vi "Measurement Logic.vi"() -> ()   [LabVIEW 2021, in "Efficiency_Channel Ganging.lvlib"]
uses:
  Efficiency_Channel Ganging.lvlib
  Measurement Configuration.ctl
  Measurement Results.ctl
  <vilib>/MeasurementLink/MeasurementLink Measurement Server/Measure Call Context/Measure Call Context.lvclass
  <instrlib>/niDCPower/nidcpower.llb/niDCPower Source Mode.ctl
  <instrlib>/niDCPower/nidcpower.llb/niDCPower Wait For Event - Event.ctl
  <instrlib>/niDCPower/nidcpower.llb/niDCPower Output Function.ctl
  shared subVIs/Triggers and Events/NIDCPower_channel_ganging - Configure Digital Edge Source Trigger.vi
  shared subVIs/Triggers and Events/NIDCPower_channel_ganging - Configure Digital Edge Measure Trigger.vi
  <vilib>/MeasurementLink/MeasurementLink Measurement Server/Measure Call Context/Accessor/Is Canceled.vi
panel:
  out "measure call context out":refnum<class "Measure Call Context.lvclass">
  in  "measure call context in":refnum<class "Measure Call Context.lvclass">
  out "measurement results":T1
  in  "measurement configuration":T2={"Source master resource name"="", "Source slave resource names"=[], "Load master resource name"="", "Load slave resource names"=[], "Source system configuration"=enum."Parallel", "Source start voltage"=6.0, "Source stop voltage"=14.0, "Source voltage sweep points"=4, "Source voltage level range"=20.0, "Source sense"=1009, "Source limit symmetry"=enum."Asymmetric", "Source current limit range"=25.0, "Source current limit low"=-0.6, "Source current limit high"=25.0, "Source transient response"=1038, "Load system configuration"=enum."Parallel", "Load start current"=1.0, "Load stop current"=50.0, "Load current sweep points/points per decade"=10, "Load sweep type"="Logarithmic", "Load current level range"=80.0, "Load sense"=1009, "Load limit symmetry"=enum."Symmetric", "Load voltage limit range"=6.0, "Load voltage limit low"=0.0, "Load voltage limit high"=inf, "Load transient response"=1038, "DUT setup time"=1.0, "Source delay"=0.005, "Aperture time"=0.005} {"Source delay" format="%#_6p"; "DUT setup time" format="%#_6p"; "Load start current" format="%#_6p"; "Source start voltage" format="%#_6p"; "Load sense" items=["Local"=1008, "Remote"=1009]; "Load transient response" items=["Slow"=1041, "Normal"=1038, "Fast"=1039, "Custom"=1042]; "Source sense" items=["Local"=1008, "Remote"=1009]; "Source transient response" items=["Slow"=1041, "Normal"=1038, "Fast"=1039, "Custom"=1042]; "Load voltage limit high" format="%#_6p"; "Load voltage limit low" format="%#_6p"; "Source current limit high" format="%#_6p"; "Source current limit low" format="%#_6p"; "Source current limit range" format="%#_6p"}
  out "error out":errorcluster
  in  "error in":errorcluster
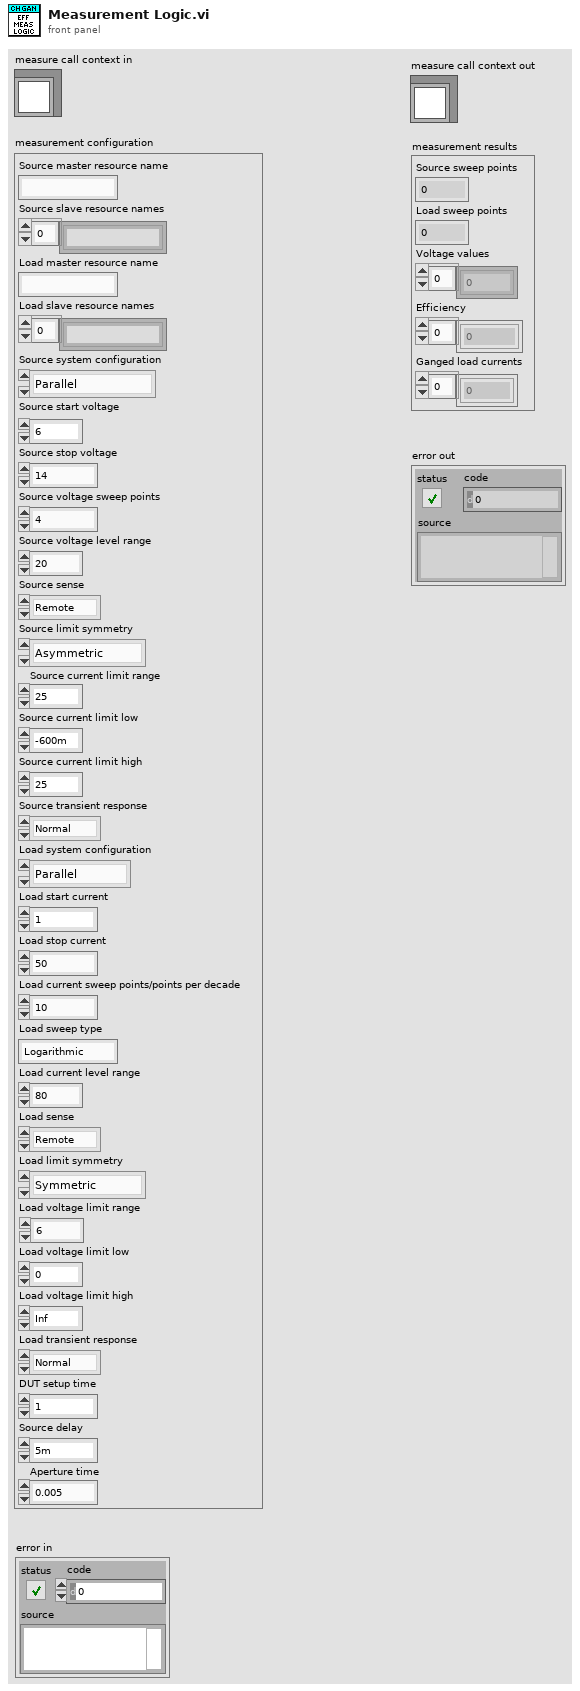
[diagram p1: front panel]
types:
  T1 = typedef "Efficiency_Channel Ganging.lvlib/Measurement Results.ctl" = cluster{"Source sweep points":i32, "Load sweep points":i32, "Voltage values":dbl[], "Efficiency":dbl[], "Ganged load currents":dbl[]}
  T2 = typedef "Efficiency_Channel Ganging.lvlib/Measurement Configuration.ctl" = cluster{"Source master resource name":string, "Source slave resource names":string[], "Load master resource name":string, "Load slave resource names":string[], "Source system configuration":enum32{"Series", "Parallel", "Manual"}, "Source start voltage":dbl, "Source stop voltage":dbl, "Source voltage sweep points":i32, "Source voltage level range":dbl, "Source sense":i32, "Source limit symmetry":enum32{"Symmetric", "Asymmetric"}, "Source current limit range":dbl, "Source current limit low":dbl, "Source current limit high":dbl, "Source transient response":i32, "Load system configuration":enum32{"Series", "Parallel", "Manual"}, "Load start current":dbl, "Load stop current":dbl, "Load current sweep points/points per decade":i32, "Load sweep type":string, "Load current level range":dbl, "Load sense":i32, "Load limit symmetry":enum32{"Symmetric", "Asymmetric"}, "Load voltage limit range":dbl, "Load voltage limit low":dbl, "Load voltage limit high":dbl, "Load transient response":i32, "DUT setup time":dbl, "Source delay":dbl, "Aperture time":dbl}
  T3 = typedef "niDCPower Output Function.ctl" = i32
  T4 = typedef "niDCPower Source Mode.ctl" = i32
  T5 = typedef "niDCPower Wait For Event - Event.ctl" = i32
  T6 = typedef "NIDCPower_channel_ganging - ctl - channel def.ctl" = cluster{"resource name":refnum<k15>, "channels":string, "Channel Mode":T7}
  T7 = typedef "NIDCPower_channel_ganging - ctl - channel mode.ctl" = enum32{"Master", "Slave", "Slave - Inverted"}
  T8 = typedef "NIDCPower_channel_ganging - ctl - ganged session.ctl" = cluster{"Ganged Config":T9, "Session List":refnum<k15>[], "Session Mode":T7[], "Channel":string[]}
  T9 = typedef "NIDCPower_channel_ganging - ctl - ganged config.ctl" = enum32{"Series", "Parallel", "Manual"}
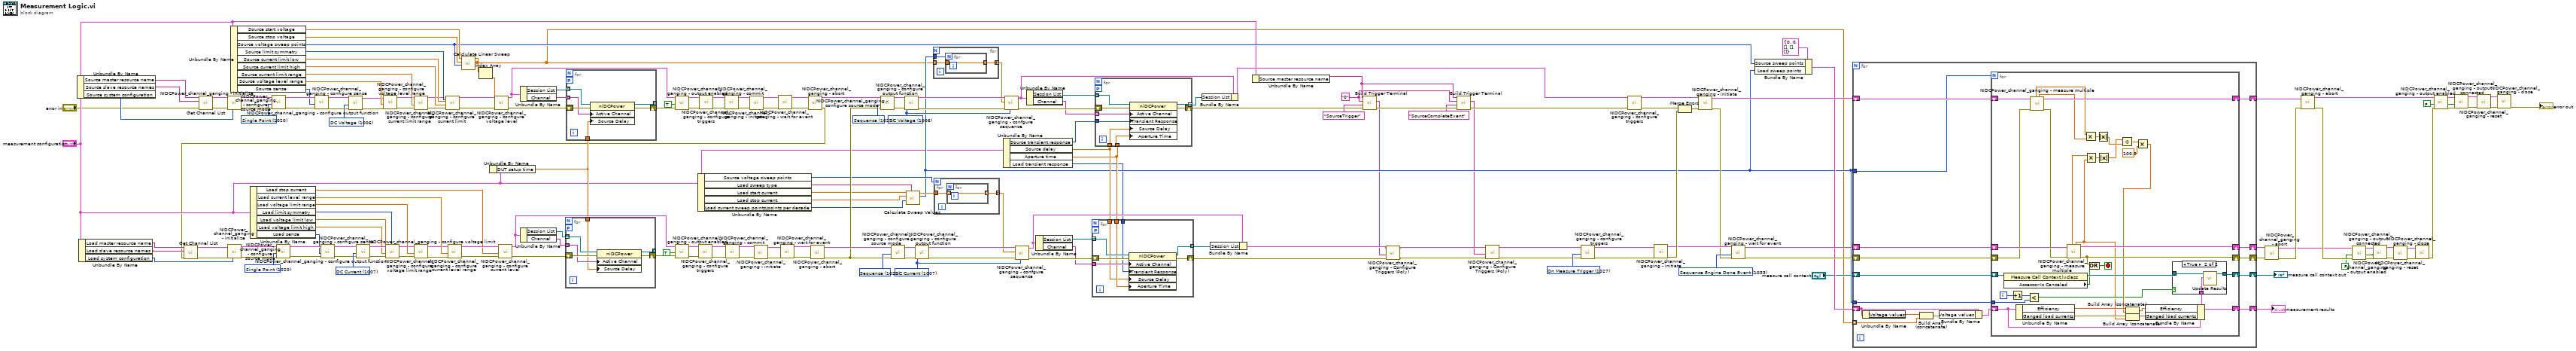
[diagram p0: block diagram]
diagram:
  w19 = "0" ("Channel Name")
  w86 = 1027 items=["Automatically after Source Complete"=1025, "On Demand"=1026, "On Measure Trigger"=1027] ("Measure When")
  w83 = T3 1006 items=["DC Voltage"=1006, "DC Current"=1007, "Pulse Voltage"=1049, "Pulse Current"=1050] ("output function")
  w88 = T4 1021 items=["Single Point"=1020, "Sequence"=1021] ("source mode")
  w89 = T4 1021 items=["Single Point"=1020, "Sequence"=1021] ("source mode")
  w64 = T3 1007 items=["DC Voltage"=1006, "DC Current"=1007, "Pulse Voltage"=1049, "Pulse Current"=1050] ("output function")
  w136 = T5 1033 items=["Source Complete Event"=1030, "Measure Complete Event"=1031, "Sequence Iteration Complete Event"=1032, "Sequence Engine Done Event"=1033, "Pulse Complete Event"=1051, "Ready For Pulse Trigger Event"=1052] ("event")
  w137 = T3 1007 items=["DC Voltage"=1006, "DC Current"=1007, "Pulse Voltage"=1049, "Pulse Current"=1050] ("output function")
  w150 = T3 1006 items=["DC Voltage"=1006, "DC Current"=1007, "Pulse Voltage"=1049, "Pulse Current"=1050] ("output function")
  w156 = FALSE ("output enabled")
  w155 = FALSE ("output enabled")
  w188 = T4 1020 items=["Single Point"=1020, "Sequence"=1021] ("source mode")
  w189 = T4 1020 items=["Single Point"=1020, "Sequence"=1021] ("source mode")
  n1 = Unbundle By Name("measurement configuration") -> ("Source master resource name"=w7:string, "Source slave resource names"=w6:string[], "Source system configuration"=w167:enum32{"Series", "Parallel", "Manual"})
  n2 = Unbundle By Name("measurement configuration") -> ("Load master resource name"=w3:string, "Load slave resource names"=w2:string[], "Load system configuration"=w166:enum32{"Series", "Parallel", "Manual"})
  n3 = call "Get Channel List.vi"("error in (no error)"="error in", "Slave resource names"=w6, "Master resouce name"=w7) -> ("error out"=w8:errorcluster, "Channel List"=w9:T6[])  [unwired: 7 in]
  n4 = call "NIDCPower_channel_ganging - initialize.vi"("Ganged Config"=w167, "error in (no error)"=w8, "Channel List"=w9) -> ("error out"=w190:errorcluster, "Ganged Session Out"=w191:T8)  [unwired: 7 in]
  n5 = Unbundle By Name("measurement configuration") -> ("Source start voltage"=w54:dbl, "Source stop voltage"=w53:dbl, "Source voltage sweep points"=w35:i32, "Source limit symmetry"=w173:enum32{"Symmetric", "Asymmetric"}, "Source current limit low"=w174:dbl, "Source current limit high"=w175:dbl, "Source current limit range"=w176:dbl, "Source voltage level range"=w177:dbl, "Source sense"=w16:i32)
  n6 = Unbundle By Name("measurement configuration") -> ("Load stop current"=w40:dbl, "Load current level range"=w168:dbl, "Load voltage limit range"=w169:dbl, "Load limit symmetry"=w172:enum32{"Symmetric", "Asymmetric"}, "Load voltage limit low"=w171:dbl, "Load voltage limit high"=w170:dbl, "Load sense"=w17:i32)
  n7 = call "NIDCPower_channel_ganging - configure source mode.vi"("error in (no error)"=w190, "source mode"=w189, "Ganged Session In"=w191) -> ("error out"=w133:errorcluster, "Ganged Session Out"=w134:T8)  [unwired: 7 in]
  n8 = call "NIDCPower_channel_ganging - configure sense.vi"("error in (no error)"=w133, "sense"=w16, "Ganged Session In"=w134) -> ("error out"=w131:errorcluster, "Ganged Session Out"=w132:T8)  [unwired: 7 in]
  n9 = call "NIDCPower_channel_ganging - configure output function.vi"("error in (no error)"=w131, "output function"=w150, "Ganged Session In"=w132) -> ("error out"=w129:errorcluster, "Ganged Session Out"=w130:T8)  [unwired: 7 in]
  n10 = call "NIDCPower_channel_ganging - configure voltage level range.vi"("error in (no error)"=w129, "voltage level range"=w177, "Ganged Session In"=w130) -> ("error out"=w146:errorcluster, "Ganged Session Out"=w149:T8)  [unwired: 7 in]
  n11 = call "NIDCPower_channel_ganging - configure current limit range.vi"("error in (no error)"=w146, "current limit range"=w176, "Ganged Session In"=w149) -> ("error out"=w145:errorcluster, "Ganged Session Out"=w148:T8)  [unwired: 7 in]
  n12 = call "NIDCPower_channel_ganging - configure current limit.vi"("Limit Symmetry"=w173, "error in (no error)"=w145, "Current limit/hi"=w175, "Current limit lo"=w174, "Ganged Session In"=w148) -> ("error out"=w144:errorcluster, "Ganged Session Out"=w147:T8)  [unwired: 5 in]
  n13 = call "Calclulate Linear Sweep.vi"("Points"=w35, "Stop level"=w53, "Start level"=w54) -> ("Values"=w18:dbl[])  [unwired: 8 in]
  n14 = Index Array(array=w18) -> (element=w55:dbl)  [unwired: 1 in]
  n15 = Unbundle By Name("measurement configuration") -> ("DUT setup time"=w39:dbl)
  n16 = call "NIDCPower_channel_ganging - configure voltage level.vi"("error in (no error)"=w144, "voltage level"=w55, "Ganged Session In"=w147) -> ("error out"=w104:errorcluster, "Ganged Session Out"=w98:T8)  [unwired: 7 in]
  n17 = Unbundle By Name(w98) -> ("Session List"=w102:refnum<k15>[], "Channel"=w101:string[])
  n18 = for {
    tunnel: [w197] -> _ mode=indexing
    shift-right: [w195] -> w103
    shift-left: w104 -> [w196]
    workers-P: _ -> [_]
    tunnel: w102 -> [w194] mode=indexing
    tunnel: w101 -> [w193] mode=indexing
    tunnel: w39 -> [w192]
    n19 = property class="niDCPower"(reference=w194, error in=w196, "Active Channel"=w193, "Source Delay"=w192) -> (reference out=w197:refnum<k15>, error out=w195:errorcluster)
  }
  n20 = call "NIDCPower_channel_ganging - output enabled.vi"("error in (no error)"=w103, "output enabled"=TRUE, "Ganged Session In"=w98) -> ("error out"=w107:errorcluster, "Ganged Session Out"=w108:T8)  [unwired: 7 in]
  n21 = Unbundle By Name("measurement configuration") -> ("Source voltage sweep points"=w41:i32, "Load sweep type"=w13:string, "Load start current"=w52:dbl, "Load stop current"=w51:dbl, "Load current sweep points/points per decade"=w50:i32)
  n22 = call "NIDCPower_channel_ganging - configure triggers.vi"("error in (no error)"=w107, "Ganged Session In"=w108) -> ("error out"=w105:errorcluster, "Ganged Session Out"=w106:T8)  [unwired: 8 in]
  n23 = call "NIDCPower_channel_ganging - commit.vi"("error in (no error)"=w105, "Ganged Session In"=w106) -> ("error out"=w114:errorcluster, "Ganged Session Out"=w113:T8)  [unwired: 8 in]
  n24 = call "NIDCPower_channel_ganging - initiate.vi"("error in (no error)"=w114, "Ganged Session In"=w113) -> ("error out"=w116:errorcluster, "Ganged Session Out"=w115:T8)  [unwired: 8 in]
  n25 = call "NIDCPower_channel_ganging - wait for event.vi"("error in (no error)"=w116, "Ganged Session in"=w115) -> ("error out"=w118:errorcluster, "Ganged Session Out"=w117:T8)  [unwired: 8 in]
  n26 = call "NIDCPower_channel_ganging - abort.vi"("error in (no error)"=w118, "Ganged Session In"=w117) -> ("error out"=w1:errorcluster, "Ganged Session Out"=w87:T8)  [unwired: 8 in]
  n27 = call "Get Channel List.vi"("error in (no error)"=w1, "Slave resource names"=w2, "Master resouce name"=w3) -> ("error out"=w5:errorcluster, "Channel List"=w4:T6[])  [unwired: 7 in]
  n28 = call "NIDCPower_channel_ganging - initialize.vi"("Ganged Config"=w166, "error in (no error)"=w5, "Channel List"=w4) -> ("error out"=w187:errorcluster, "Ganged Session Out"=w186:T8)  [unwired: 7 in]
  n29 = call "NIDCPower_channel_ganging - configure source mode.vi"("error in (no error)"=w187, "source mode"=w188, "Ganged Session In"=w186) -> ("error out"=w127:errorcluster, "Ganged Session Out"=w128:T8)  [unwired: 7 in]
  n30 = call "NIDCPower_channel_ganging - configure sense.vi"("error in (no error)"=w127, "sense"=w17, "Ganged Session In"=w128) -> ("error out"=w125:errorcluster, "Ganged Session Out"=w126:T8)  [unwired: 7 in]
  n31 = call "NIDCPower_channel_ganging - configure output function.vi"("error in (no error)"=w125, "output function"=w137, "Ganged Session In"=w126) -> ("error out"=w184:errorcluster, "Ganged Session Out"=w185:T8)  [unwired: 7 in]
  n32 = call "NIDCPower_channel_ganging - configure voltage limit.vi"("Limit Symmetry"=w172, "error in (no error)"=w184, "voltage limit/hi"=w170, "voltage limit lo"=w171, "Ganged Session In"=w185) -> ("error out"=w142:errorcluster, "Ganged Session Out"=w143:T8)  [unwired: 5 in]
  n33 = call "NIDCPower_channel_ganging - configure voltage limit range.vi"("error in (no error)"=w142, "voltage level range"=w169, "Ganged Session In"=w143) -> ("error out"=w140:errorcluster, "Ganged Session Out"=w141:T8)  [unwired: 7 in]
  n34 = call "NIDCPower_channel_ganging - configure current level range.vi"("error in (no error)"=w140, "current level range"=w168, "Ganged Session In"=w141) -> ("error out"=w138:errorcluster, "Ganged Session Out"=w139:T8)  [unwired: 7 in]
  n35 = call "NIDCPower_channel_ganging - configure current level.vi"("error in (no error)"=w138, "current level"=w40, "Ganged Session In"=w139) -> ("error out"=w100:errorcluster, "Ganged Session Out"=w97:T8)  [unwired: 7 in]
  n36 = Unbundle By Name(w97) -> ("Session List"=w96:refnum<k15>[], "Channel"=w95:string[])
  n37 = for {
    tunnel: [w203] -> _ mode=indexing
    shift-right: [w201] -> w99
    shift-left: w100 -> [w202]
    workers-P: _ -> [_]
    tunnel: w96 -> [w200] mode=indexing
    tunnel: w95 -> [w199] mode=indexing
    tunnel: w39 -> [w198]
    n38 = property class="niDCPower"(reference=w200, error in=w202, "Active Channel"=w199, "Source Delay"=w198) -> (reference out=w203:refnum<k15>, error out=w201:errorcluster)
  }
  n39 = call "NIDCPower_channel_ganging - output enabled.vi"("error in (no error)"=w99, "output enabled"=TRUE, "Ganged Session In"=w97) -> ("error out"=w111:errorcluster, "Ganged Session Out"=w112:T8)  [unwired: 7 in]
  n40 = call "NIDCPower_channel_ganging - configure triggers.vi"("error in (no error)"=w111, "Ganged Session In"=w112) -> ("error out"=w109:errorcluster, "Ganged Session Out"=w110:T8)  [unwired: 8 in]
  n41 = call "NIDCPower_channel_ganging - commit.vi"("error in (no error)"=w109, "Ganged Session In"=w110) -> ("error out"=w123:errorcluster, "Ganged Session Out"=w124:T8)  [unwired: 8 in]
  n42 = call "NIDCPower_channel_ganging - initiate.vi"("error in (no error)"=w123, "Ganged Session In"=w124) -> ("error out"=w121:errorcluster, "Ganged Session Out"=w122:T8)  [unwired: 8 in]
  n43 = call "NIDCPower_channel_ganging - wait for event.vi"("error in (no error)"=w121, "Ganged Session in"=w122) -> ("error out"=w119:errorcluster, "Ganged Session Out"=w120:T8)  [unwired: 8 in]
  n44 = call "NIDCPower_channel_ganging - abort.vi"("error in (no error)"=w119, "Ganged Session In"=w120) -> ("error out"=w56:errorcluster, "Ganged Session Out"=w90:T8)  [unwired: 8 in]
  n45 = call "NIDCPower_channel_ganging - configure source mode.vi"("error in (no error)"=w56, "source mode"=w88, "Ganged Session In"=w87) -> ("error out"=w91:errorcluster, "Ganged Session Out"=w92:T8)  [unwired: 7 in]
  n46 = call "NIDCPower_channel_ganging - configure source mode.vi"("error in (no error)"=w56, "source mode"=w89, "Ganged Session In"=w90) -> ("error out"=w94:errorcluster, "Ganged Session Out"=w93:T8)  [unwired: 7 in]
  n47 = call "NIDCPower_channel_ganging - configure output function.vi"("error in (no error)"=w91, "output function"=w83, "Ganged Session In"=w92) -> ("error out"=w84:errorcluster, "Ganged Session Out"=w85:T8)  [unwired: 7 in]
  n48 = call "Calculate Sweep Values.vi"("Sweep type"=w13, "Points"=w50, "Stop level"=w51, "Start level"=w52) -> ("Sweep points"=w34:i32, "Sweep values"=w49:dbl[])  [unwired: 5 in, 1 out]
  n49 = call "NIDCPower_channel_ganging - configure output function.vi"("error in (no error)"=w94, "output function"=w64, "Ganged Session In"=w93) -> ("error out"=w65:errorcluster, "Ganged Session Out"=w66:T8)  [unwired: 7 in]
  n50 = for {
    tunnel: w18 -> [w206] mode=indexing
    tunnel: [w205] -> w47 mode=concatenating
    tunnel: w34 -> [w204]
    n51 = for {
      N: w204 -> [_]
      tunnel: w206 -> [w207]
      tunnel: [w207] -> w205 mode=indexing
    }
  }
  n52 = for {
    N: w41 -> [_]
    tunnel: w49 -> [w209]
    tunnel: [w208] -> w48 mode=concatenating
    n53 = for {
      tunnel: w209 -> [w210] mode=indexing
      tunnel: [w210] -> w208 mode=indexing
    }
  }
  n54 = Unbundle By Name("measurement configuration") -> ("Source transient response"=w15:i32, "Source delay"=w37:dbl, "Aperture time"=w38:dbl, "Load transient response"=w14:i32)
  n55 = call "NIDCPower_channel_ganging - confgure sequence.vi"("output function"=w83, "error in (no error)"=w84, "Values"=w47, "Ganged Session In"=w85) -> ("error out"=w82:errorcluster, "Ganged Session Out"=w62:T8)  [unwired: 6 in]
  n56 = call "NIDCPower_channel_ganging - confgure sequence.vi"("output function"=w64, "error in (no error)"=w65, "Values"=w48, "Ganged Session In"=w66) -> ("error out"=w63:errorcluster, "Ganged Session Out"=w57:T8)  [unwired: 6 in]
  n57 = Unbundle By Name(w62) -> ("Session List"=w181:refnum<k15>[], "Channel"=w61:string[])
  n58 = Unbundle By Name(w57) -> ("Session List"=w60:refnum<k15>[], "Channel"=w59:string[])
  n59 = for {
    tunnel: [w218] -> w58 mode=indexing
    shift-right: [w216] -> w26
    shift-left: w63 -> [w217]
    workers-P: _ -> [_]
    tunnel: w60 -> [w215] mode=indexing
    tunnel: w59 -> [w214] mode=indexing
    tunnel: w38 -> [w213]
    tunnel: w37 -> [w212]
    tunnel: w14 -> [w211]
    n60 = property class="niDCPower"(reference=w215, error in=w217, "Active Channel"=w214, "Transient Response"=w211, "Source Delay"=w212, "Aperture Time"=w213) -> (reference out=w218:refnum<k15>, error out=w216:errorcluster)
  }
  n61 = for {
    tunnel: [w226] -> w180 mode=indexing
    shift-right: [w224] -> w21
    shift-left: w82 -> [w225]
    workers-P: _ -> [_]
    tunnel: w181 -> [w223] mode=indexing
    tunnel: w61 -> [w222] mode=indexing
    tunnel: w37 -> [w220]
    tunnel: w38 -> [w221]
    tunnel: w15 -> [w219]
    n62 = property class="niDCPower"(reference=w223, error in=w225, "Active Channel"=w222, "Transient Response"=w219, "Source Delay"=w220, "Aperture Time"=w221) -> (reference out=w226:refnum<k15>, error out=w224:errorcluster)
  }
  n63 = Bundle By Name(cluster=w62, "Session List"=w180) -> (w46:T8)
  n64 = Bundle By Name(cluster=w57, "Session List"=w58) -> (w27:T8)
  n65 = Unbundle By Name("measurement configuration") -> ("Source master resource name"=w20:string)
  n66 = call "Build Trigger Terminal.vi"("error in (no error)"=w21, "Trigger/Event Name"="SourceTrigger", "Channel Name"=w19, "Resource Name"=w20) -> ("error out"=w45:errorcluster, "Terminal Name"=w12:string)  [unwired: 6 in]
  n67 = call-poly "NIDCPower_channel_ganging - Configure Triggers (Poly).vi"("error in (no error)"=w26, "output terminal"=w12, "Ganged Session in"=w27) -> ("error out"=w22:errorcluster, "Ganged Session out"=w23:T8)  [unwired: 7 in]
  n68 = call "Build Trigger Terminal.vi"("error in (no error)"=w45, "Trigger/Event Name"="SourceCompleteEvent", "Channel Name"=w19, "Resource Name"=w20) -> ("error out"=w44:errorcluster, "Terminal Name"=w11:string)  [unwired: 6 in]
  n69 = call-poly "NIDCPower_channel_ganging - Configure Triggers (Poly).vi"("error in (no error)"=w22, "output terminal"=w11, "Ganged Session in"=w23) -> ("error out"=w24:errorcluster, "Ganged Session out"=w25:T8)  [unwired: 7 in]
  n70 = call "NIDCPower_channel_ganging - configure triggers.vi"("error in (no error)"=w24, "Measure When"=w86, "Ganged Session In"=w25) -> ("error out"=w178:errorcluster, "Ganged Session Out"=w179:T8)  [unwired: 7 in]
  n71 = call "NIDCPower_channel_ganging - configure triggers.vi"("error in (no error)"=w44, "Ganged Session In"=w46) -> ("error out"=w152:errorcluster, "Ganged Session Out"=w153:T8)  [unwired: 8 in]
  n72 = call "NIDCPower_channel_ganging - initiate.vi"("error in (no error)"=w178, "Ganged Session In"=w179) -> ("error out"=w151:errorcluster, "Ganged Session Out"=w135:T8)  [unwired: 8 in]
  n73 = Merge Errors(w152, w151) -> (w154:errorcluster)
  n74 = call "NIDCPower_channel_ganging - initiate.vi"("error in (no error)"=w154, "Ganged Session In"=w153) -> ("error out"=w81:errorcluster, "Ganged Session Out"=w68:T8)  [unwired: 8 in]
  n75 = call "NIDCPower_channel_ganging - wait for event.vi"("error in (no error)"=w81, "event"=w136, "Ganged Session in"=w135) -> ("error out"=w72:errorcluster, "Ganged Session Out"=w70:T8)  [unwired: 7 in]
  n76 = Bundle By Name(cluster=T1 {"Source sweep points"=0, "Load sweep points"=0, "Voltage values"=[], "Efficiency"=[], "Ganged load currents"=[]} ("Measurement Results"), "Source sweep points"=w35, "Load sweep points"=w34) -> (w36:T1)
  n77 = for {
    shift-right: [w241] -> w71
    shift-left: w72 -> [w242]
    shift-right: [w239] -> w69
    shift-left: w70 -> [w240]
    shift-right: [w237] -> w67
    shift-left: w68 -> [w238]
    tunnel: w34 -> [w236]
    shift-right: [w234] -> w29
    shift-left: "measure call context in" -> [w235]
    shift-right: [w233] -> w31
    shift-left: w36 -> [w228]
    tunnel: w34 -> [w232]
    tunnel: w18 -> [w227] mode=indexing
    n78 = Unbundle By Name(w228) -> ("Voltage values"=w231:dbl[])
    n79 = Build Array (concatenate)(w231, w227) -> (w230:dbl[])
    n80 = Bundle By Name(cluster=w228, "Voltage values"=w230) -> (w229:T1)
    n81 = for {
      N: w236 -> [_]
      shift-right: [w264] -> w241
      shift-left: w242 -> [w273]
      shift-right: [w274] -> w239
      shift-left: w240 -> [w275]
      shift-right: [w270] -> w237
      shift-left: w238 -> [w271]
      shift-right: [w267] -> w234
      shift-left: w235 -> [w269]
      shift-right: [w254] -> w233
      shift-left: w229 -> [w258]
      tunnel: w232 -> [w250]
      i -> [w251]
      stop <- w266 stop-if-true
      n82 = property class="Measure Call Context.lvclass"(reference=w269) -> (reference out=w268:refnum<class "Measure Call Context.lvclass">, "Accessor:Is Canceled"=w265:bool)  [unwired: 1 in, 1 out]
      n83 = Increment(x=w251) -> (x+1=w252:i32)
      n84 = Unbundle By Name(w258) -> ("Efficiency"=w263:dbl[], "Ganged load currents"=w257:dbl[])
      n85 = Less?(x=w252, y=w250) -> (x < y?=w249:bool)
      n86 = call "NIDCPower_channel_ganging - measure multiple.vi"("error in (no error)"=w273, "Ganged Session In"=w271) -> ("error out"=w272:errorcluster, "Ganged Session Out"=w270:T8, "ganged current measurement"=w246:dbl, "ganged voltage measurement"=w245:dbl)  [unwired: 2 in, 4 out]
      n87 = call "NIDCPower_channel_ganging - measure multiple.vi"("error in (no error)"=w272, "Ganged Session In"=w275) -> ("error out"=w264:errorcluster, "Ganged Session Out"=w274:T8, "ganged current measurement"=w247:dbl, "ganged voltage measurement"=w248:dbl)  [unwired: 2 in, 4 out]
      n88 = Multiply(x=w245, y=w246) -> (x*y=w260:dbl)
      n89 = Multiply(x=w248, y=w247) -> (x*y=w259:dbl)
      n90 = Compound Arithmetic op=OR(w264, w265) -> (w266:bool)
      n91 = Absolute Value(x=w260) -> (abs(x)=w244:dbl)
      n92 = Absolute Value(x=w259) -> (abs(x)=w243:dbl)
      n93 = Divide(x=w243, y=w244) -> (x/y=w262:dbl)
      n94 = Build Array (concatenate)(w257, w247) -> (w255:dbl[])
      n95 = Multiply(x=w262, y=100.0) -> (x*y=w253:dbl)
      n96 = Build Array (concatenate)(w263, w253) -> (w256:dbl[])
      n97 = Bundle By Name(cluster=w258, "Efficiency"=w256, "Ganged load currents"=w255) -> (w254:T1)
      n98 = case shown="True" w249 {
        tunnel: w254 -> [_ w279]
        tunnel: w268 -> [w276 w278]
        tunnel: [w276 w277] -> w267
        frame False {
        }
        frame True {
          n99 = call <vilib>:"Update Results.vi"("measurement results"=w279, "measure call context in"=w278) -> ("measure call context out"=w277:refnum<class "Measure Call Context.lvclass">)  [unwired: 8 in, 1 out]
        }
      }
    }
  }
  "measurement results" <- w31
  "measure call context out" <- w29
  n100 = call "NIDCPower_channel_ganging - abort.vi"("error in (no error)"=w71, "Ganged Session In"=w69) -> ("error out"=w165:errorcluster, "Ganged Session Out"=w161:T8)  [unwired: 8 in]
  n101 = call "NIDCPower_channel_ganging - abort.vi"("error in (no error)"=w165, "Ganged Session In"=w67) -> ("error out"=w164:errorcluster, "Ganged Session Out"=w157:T8)  [unwired: 8 in]
  n102 = call "NIDCPower_channel_ganging - output enabled.vi"("error in (no error)"=w164, "output enabled"=w156, "Ganged Session In"=w161) -> ("error out"=w162:errorcluster, "Ganged Session Out"=w163:T8)  [unwired: 7 in]
  n103 = call "NIDCPower_channel_ganging - output connected.vi"("error in (no error)"=w162, "output enabled"=w156, "Ganged Session In"=w163) -> ("error out"=w80:errorcluster, "Ganged Session Out"=w79:T8)  [unwired: 7 in]
  n104 = call "NIDCPower_channel_ganging - reset.vi"("error in (no error)"=w80, "Ganged Session In"=w79) -> ("error out"=w77:errorcluster, "Ganged Session Out"=w78:T8)  [unwired: 8 in]
  n105 = call "NIDCPower_channel_ganging - close.vi"("error in (no error)"=w77, "Ganged Session In"=w78) -> ("error out"=w158:errorcluster)  [unwired: 9 in]
  n106 = call "NIDCPower_channel_ganging - output enabled.vi"("error in (no error)"=w158, "output enabled"=w155, "Ganged Session In"=w157) -> ("error out"=w160:errorcluster, "Ganged Session Out"=w159:T8)  [unwired: 7 in]
  n107 = call "NIDCPower_channel_ganging - output connected.vi"("error in (no error)"=w160, "output enabled"=w155, "Ganged Session In"=w159) -> ("error out"=w75:errorcluster, "Ganged Session Out"=w76:T8)  [unwired: 7 in]
  n108 = call "NIDCPower_channel_ganging - reset.vi"("error in (no error)"=w75, "Ganged Session In"=w76) -> ("error out"=w73:errorcluster, "Ganged Session Out"=w74:T8)  [unwired: 8 in]
  n109 = call "NIDCPower_channel_ganging - close.vi"("error in (no error)"=w73, "Ganged Session In"=w74) -> ("error out"=→"error out":errorcluster)  [unwired: 9 in]
